vi "Report_Tables.vi"(4 "Measurement System":i32, 5 "Column Width":dbl[](array[numeric]) format="%.2f", 6 "text data":string[][](array[string]), 7 "show grid lines":bool, 8 "error in (no error)":errorcluster, 9 "row headers":string[](array[string]), 10 "column headers":string[](array[string]), 11 "report in":T1) -> (0 "error out":errorcluster, 3 "report out":T1)   [LabVIEW 2020]
uses:
  <vilib>/Utility/NIReport.llb/NI_report.lvclass
  <vilib>/Utility/NIReport.llb/Generate Report Object Reference.ctl
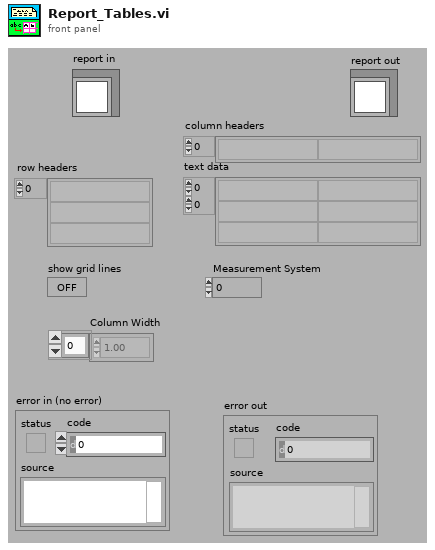
[diagram p1: front panel]
types:
  T1 = typedef "Generate Report Object Reference.ctl" = refnum<class "NI_report.lvclass">
  T2 = typedef "Generate Report Data Members.ctl" = cluster{"Title Text":string, "Header Text":string, "Body Text":string, "Footer Text":string, "Image List":path[], "NIReports.Report":refnum<k7>, "Report Type":enum16{"Standard Report", "HTML", "Word", "Excel"}, "Font Tag":string, "Word._Application":refnum<k7>, "Word._Document":refnum<k7>, "Word.Documents":refnum<k7>, "Word.InlineShapes":refnum<k7>, "Word.Tables":refnum<k7>, "Excel._Application":refnum<k7>, "Excel._Workbook":refnum<k7>, "Excel._Worksheet":refnum<k7>, "Excel.Sheets":refnum<k7>, "Excel.Shapes":refnum<k7>, "font":T3, "application directory":path, "application already open":bool, "from template?":bool}
  T3 = typedef "font.ctl" = cluster{"font name":string, "font size":dbl, "bold":u16, "italic":u16, "underline":u16, "strike through":u16, "font color":u32}
  T4 = typedef "Generate Report Object Reference.ctl" = refnum<k1>
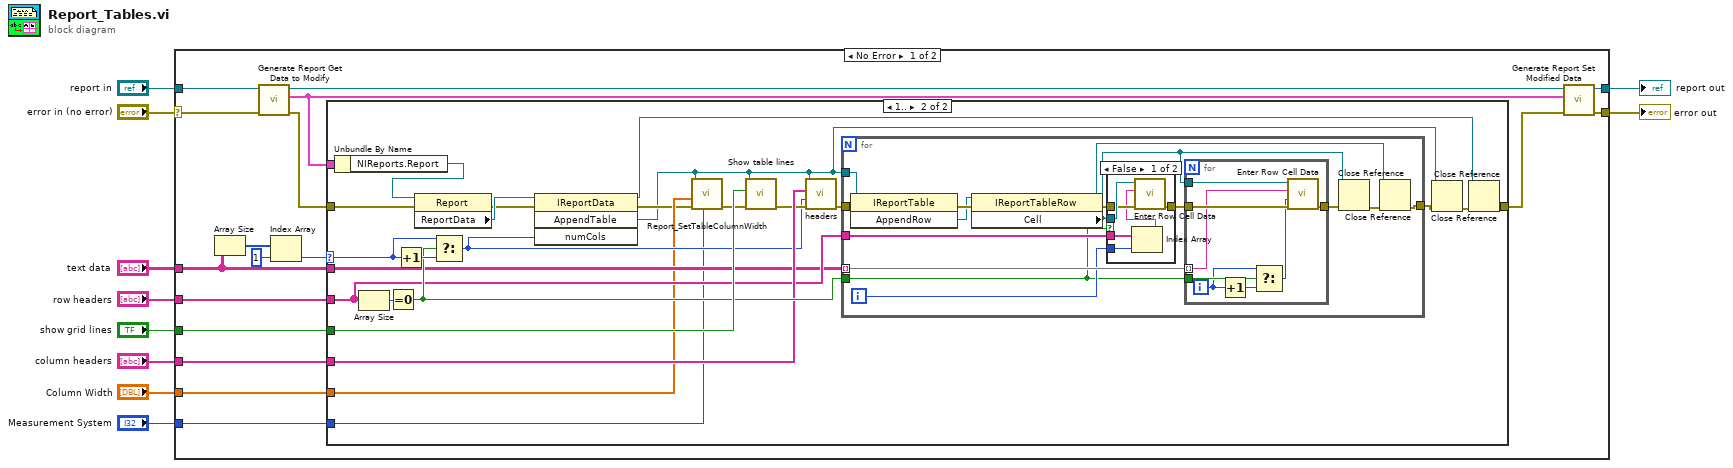
[diagram p0: block diagram]
diagram:
  n1 = case shown="No Error" "error in (no error)" {
    selector: "error in (no error)" -> [w11 w84]
    tunnel: "show grid lines" -> [w26 _]
    tunnel: "column headers" -> [w25 _]
    tunnel: "row headers" -> [w24 _]
    tunnel: "text data" -> [w23 _]
    tunnel: "report in" -> [w20 _]
    tunnel: [w19 _] -> w5
    tunnel: "Measurement System" -> [w18 _]
    tunnel: [w13 w84] -> w3
    tunnel: "Column Width" -> [w12 _]
    frame No Error {
      n2 = Array Size(array=w23) -> (size(s)=w27:i32[])
      n3 = call <vilib>:"Generate Report Get Data to Modify.vi"("error in (no error)"=w11, "report in"=w20) -> ("error out"=w21:errorcluster, "data"=w16:T2, "report out"=w22:T4)  [unwired: 2 in, 1 out]
      n4 = Index Array(array=w27, index=1 ("Index")) -> (element=w14:i32)
      n5 = case shown="1.." w14 {
        selector: w14 -> [_ w30]
        tunnel: w26 -> [_ w51]
        tunnel: w25 -> [_ w46]
        tunnel: w24 -> [_ w45]
        tunnel: w23 -> [_ w44]
        tunnel: w21 -> [w28 w42]
        tunnel: w16 -> [_ w41]
        tunnel: w12 -> [_ w38]
        tunnel: w18 -> [_ w29]
        tunnel: [w28 w32] -> w17
        frame 0, Default {
        }
        frame 1.. {
          n6 = Unbundle By Name(w41) -> ("NIReports.Report"=w43:refnum<k7>)
          n7 = Array Size(array=w45) -> (size(s)=w50:i32)
          n8 = Equal To 0?(x=w50) -> (x = 0?=w47:bool)
          n9 = Increment(x=w30) -> (x+1=w48:i32)
          n10 = property class="Report"(reference=w43, error in=w42) -> (error out=w52:errorcluster, "ReportData"=w53:refnum<k7>)  [unwired: 1 out]
          n11 = Select(t=w30, s=w47, f=w48) -> (s? t:f=w39:i32)
          n12 = invoke class="IReportData" method="AppendTable"(reference=w53, error in=w52, "numCols"=w39) -> (reference out=w31:refnum<k7>, error out=w37:errorcluster, "AppendTable"=w35:refnum<k7>)  [unwired: 1 in, 1 out]
          n13 = call "Report_SetTableColumnWidth.vi"("MeasurementSystem"=w29, "error in"=w37, "Column Width"=w38, "AppendTable"=w35) -> ("error out"=w36:errorcluster)  [unwired: 7 in]
          n14 = call <vilib>:"Show table lines.vi"("error in"=w36, "Show Table Lines"=w51, "AppendTable"=w35) -> ("error out"=w40:errorcluster)  [unwired: 8 in]
          n15 = call <vilib>:"headers.vi"("error in"=w40, "Number of Columns"=w39, "Column Headers"=w46, "AppendTable"=w35) -> ("error out"=w49:errorcluster)  [unwired: 7 in]
          n16 = for {
            tunnel: w44 -> [w68] mode=indexing
            tunnel: w35 -> [w65]
            tunnel: w49 -> [w66]
            tunnel: w45 -> [w64]
            tunnel: w47 -> [w60]
            tunnel: [w56] -> w34
            i -> [w63]
            n17 = invoke class="IReportTable" method="AppendRow"(reference=w65, error in=w66) -> (error out=w67:errorcluster, "AppendRow"=w59:refnum<k7>)  [unwired: 1 in, 1 out]
            n18 = property class="IReportTableRow"(reference=w59, error in=w67) -> (reference out=w54:refnum<k7>, error out=w62:errorcluster, "Cell"=w55:refnum<k7>)
            n19 = case shown="False" w60 {
              tunnel: w64 -> [w74 _]
              tunnel: w63 -> [w73 _]
              tunnel: w55 -> [w72 _]
              tunnel: w62 -> [w71 w75]
              tunnel: [w70 w75] -> w61
              frame False {
                n20 = Index Array(array=w74, index=w73) -> (element=w69:string)
                n21 = call <vilib>:"Enter Row Cell Data.vi"("error in (no error)"=w71, "Text"=w69, "Cell"=w72) -> ("error out"=w70:errorcluster)  [unwired: 8 in]
              }
              frame True {
              }
            }
            n22 = for {
              tunnel: w55 -> [w80]
              tunnel: w68 -> [w82] mode=indexing
              tunnel: w61 -> [w83]
              tunnel: [w81] -> w57
              tunnel: w60 -> [w78]
              i -> [w77]
              n23 = Increment(x=w77) -> (x+1=w79:i32)
              n24 = Select(t=w77, s=w78, f=w79) -> (s? t:f=w76:i32)
              n25 = call <vilib>:"Enter Row Cell Data.vi"("error in (no error)"=w83, "Row Index"=w76, "Text"=w82, "Cell"=w80) -> ("error out"=w81:errorcluster)  [unwired: 7 in]
            }
            n26 = Close Reference(reference=w55, error in (no error)=w57) -> (error out=w58:errorcluster)
            n27 = Close Reference(reference=w54, error in (no error)=w58) -> (error out=w56:errorcluster)
          }
          n28 = Close Reference(reference=w35, error in (no error)=w34) -> (error out=w33:errorcluster)
          n29 = Close Reference(reference=w31, error in (no error)=w33) -> (error out=w32:errorcluster)
        }
      }
      n30 = call <vilib>:"Generate Report Set Modified Data.vi"("error in (no error)"=w17, "data"=w16, "report in"=w22) -> ("error out"=w13:errorcluster, "report out"=w19:T4)  [unwired: 3 in]
    }
    frame Error {
    }
  }
  "report out" <- w5
  "error out" <- w3
